vi "fileCheck.vi"(0 "fileName":string, 5 "netPath":path, 7 "status":refnum<vi>, 9 "testCount":i32, 11 "basicPath":path) -> (4 "fileName Out":string, 6 "布尔":bool)   [LabVIEW 2011]
uses:
  <vilib>/regexp/Match Regular Expression.xnode
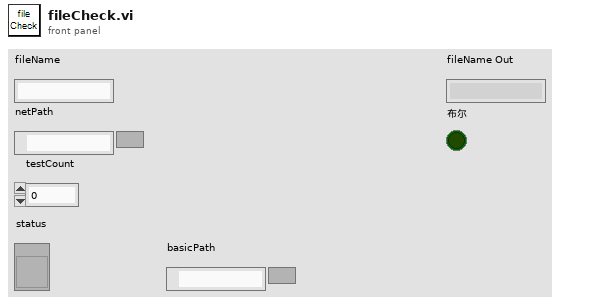
[diagram p1: front panel]
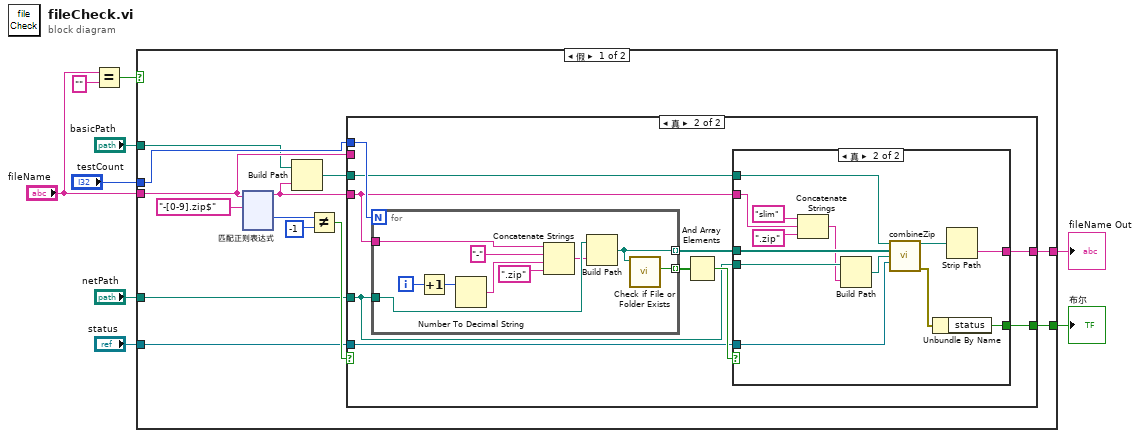
[diagram p0: block diagram]
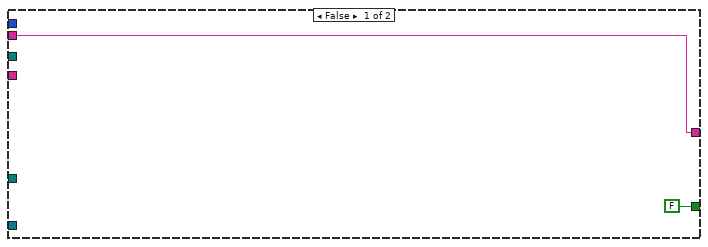
[diagram p2: hidden frame]
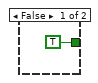
[diagram p3: hidden frame]
diagram:
  n1 = Equal?(x="fileName", y="") -> (x = y?=w5:bool)
  n2 = case shown="假" w5 {
    selector: w5 -> [_ w170]
    tunnel: "netPath" -> [w18 _]
    tunnel: "testCount" -> [w17 _]
    tunnel: "fileName" -> [w16 _]
    tunnel: [w15 w170] -> w3
    tunnel: [w14 _] -> w4
    tunnel: "status" -> [w13 _]
    tunnel: "basicPath" -> [w12 _]
    frame False {
      n3 = xnode "匹配正则表达式"("输入字符串"=w16, "正则表达式"="-[0-9].zip$") -> ("匹配之前"=w11:string, "匹配后偏移量"=w21:i32)  [unwired: 4 in, 3 out]
      n4 = Build Path(base path=w12, name or relative path=w11) -> (appended path=w10:path)
      n5 = Not Equal?(x=w21, y=-1) -> (x != y?=w19:bool)
      n6 = case shown="真" w19 {
        tunnel: w11 -> [_ w30]
        tunnel: w16 -> [w24 _]
        tunnel: w18 -> [_ w29]
        tunnel: w17 -> [_ w34]
        tunnel: [FALSE ("status") w28] -> w15
        tunnel: [w24 w25] -> w14
        tunnel: w13 -> [_ w27]
        tunnel: w10 -> [_ w26]
        frame False {
        }
        frame True {
          n7 = for {
            N: w34 -> [_]
            tunnel: w29 -> [w58]
            tunnel: [w53] -> w31 mode=indexing
            tunnel: [w52] -> w33 mode=indexing
            tunnel: w30 -> [w49]
            i -> [w51]
            n8 = Increment(x=w51) -> (x+1=w50:i32)
            n9 = Number To Decimal String(number=w50) -> (decimal integer string=w57:string)  [unwired: 1 in]
            n10 = Concatenate Strings(w49, "-" ("字符串"), w57, ".zip" ("字符串")) -> (w55:string)
            n11 = Build Path(base path=w58, name or relative path=w55) -> (appended path=w53:path)
            n12 = call <vilib>:"Check if File or Folder Exists.vi"("path"=w53) -> ("file or folder exists?"=w52:bool)  [unwired: 8 in, 2 out]
          }
          n13 = And Array Elements(Boolean array=w33) -> (logical AND=w32:bool)
          n14 = case shown="真" w32 {
            tunnel: [TRUE ("status") w40] -> w28
            tunnel: w31 -> [_ w48]
            tunnel: w30 -> [_ w47]
            tunnel: w29 -> [_ w44]
            tunnel: w27 -> [_ w39]
            tunnel: w26 -> [_ w38]
            tunnel: [_ w36] -> w25
            frame False {
            }
            frame True {
              n15 = Concatenate Strings("slim" ("字符串"), w47, ".zip" ("字符串")) -> (w43:string)
              n16 = Build Path(base path=w44, name or relative path=w43) -> (appended path=w42:path)
              n17 = call "combineZip.vi"("basicPath"=w38, "zipArray"=w48, "combinedZip"=w42, "status"=w39) -> ("combinedZip out"=w37:path, "error IO"=w41:errorcluster)  [unwired: 10 in]
              n18 = Unbundle By Name(w41) -> ("status"=w40:bool)
              n19 = Strip Path(path=w37) -> (name=w36:string)  [unwired: 1 out]
            }
          }
        }
      }
    }
    frame True {
    }
  }
  "fileName Out" <- w4
  "布尔" <- w3
